vi "数据补传对话框.vi"(11 "起始时间":timestamp) -> (1 "结束时间输出":timestamp, 2 "起始时间输出":timestamp, 3 "输出":bool=TRUE)   [LabVIEW 2016, in "数据传输系统-06.lvlib"]
panel:
  in  "结束时间":timestamp
  in  "取消":bool
  in  "确定":bool
  # "数据补传时间选择"
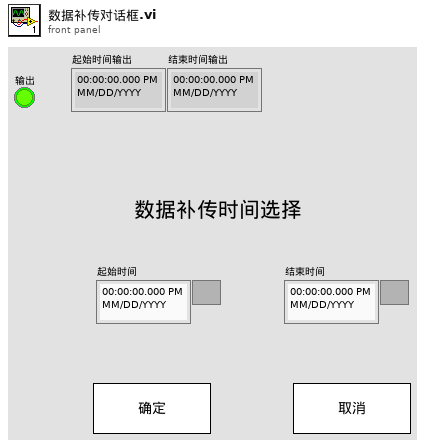
[diagram p1: front panel]
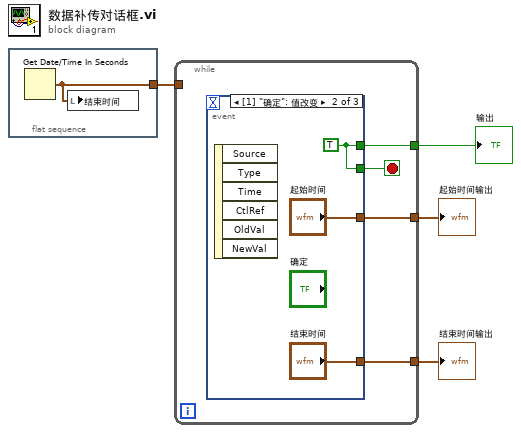
[diagram p0: block diagram]
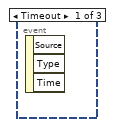
[diagram p2: hidden frame]
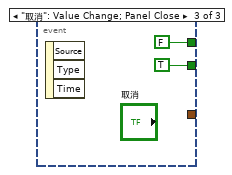
[diagram p3: hidden frame]
diagram:
  n1 = flat-sequence {
    tunnel: [w5] -> w1
    frame #0 {
      n2 = Get Date/Time In Seconds() -> (seconds since 1Jan1904=w5:timestamp)
      n3 = local write "结束时间"(w5) -> ()
    }
  }
  n4 = while {
    tunnel: [w9] -> w4
    tunnel: [w7] -> w3
    tunnel: [w6] -> w2
    tunnel: w1 -> [_]
    stop <- w8 stop-if-true
    n5 = event shown="[1] \"确定\": 值改变" {
      selector: _ -> [_ _ _]
      dyn-events: _ -> [_ _ _]
      timeout: _ -> [_ _ _]
      tunnel: [_ w12 FALSE] -> w9
      tunnel: [_ w12 TRUE] -> w8
      tunnel: [_ "起始时间" _] -> w7
      tunnel: [_ "结束时间" _] -> w6
      event Timeout {
        n6 = event-data() -> ()  [unwired: 1 in, 3 out]
      }
      event "确定": Value Change {
        w12 = TRUE
        n7 = event-data() -> ()  [unwired: 1 in, 6 out]
      }
      event "取消": Value Change; Panel Close {
        n8 = event-data() -> ()  [unwired: 1 in, 3 out]
      }
    }
  }
  "输出" <- w4
  "起始时间输出" <- w3
  "结束时间输出" <- w2
